vi "computeSetpoints.vi"(9 "Mdot":dbl, 10 "OffCentre":dbl, 11 "MFCsIn":T1[](array[typedef])) -> (1 "InactiveMFCs 2":T1[](array[typedef]), 3 "ActiveMFCs":T1[](array[typedef]))   [LabVIEW 2016]
uses:
  MFCdescription.ctl
  MFCcapability.ctl
panel:
  out "mDotTotal":dbl
  out "mDots":dbl[](array[numeric])
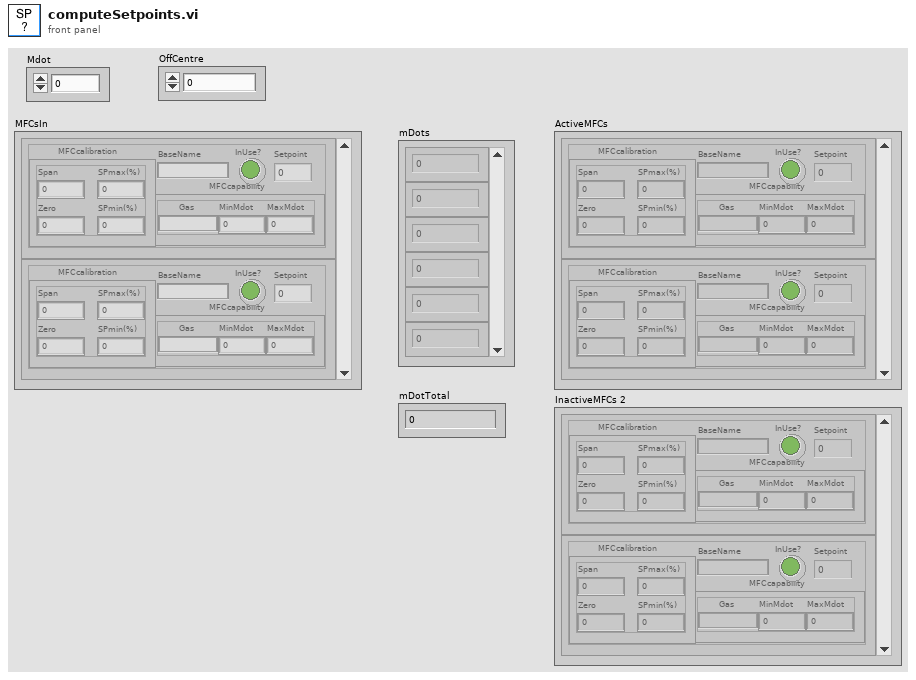
[diagram p1: front panel]
types:
  T1 = typedef "MFCdescription.ctl" = cluster{"BaseName":string, "MFCcalibration":cluster{"Span":dbl, "Zero":dbl, "SPmin(%)":dbl, "SPmax(%)":dbl}, "MFCcapability":T2, "InUse?":bool, "Setpoint":dbl}
  T2 = typedef "MFCcapability.ctl" = cluster{"Gas":string, "MinMdot":dbl, "MaxMdot":dbl}
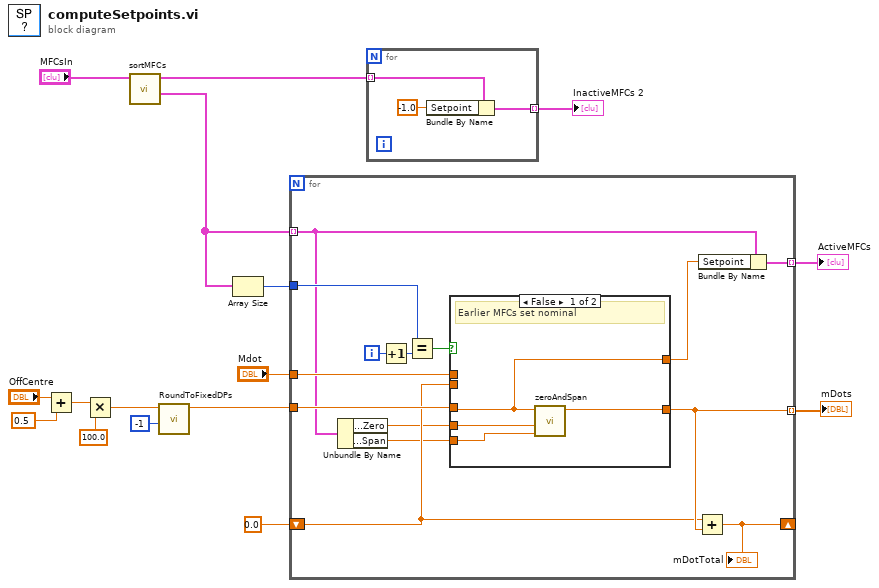
[diagram p0: block diagram]
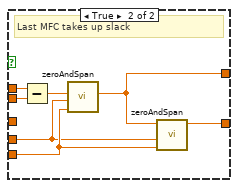
[diagram p2: hidden frame]
diagram:
  n1 = Add(x="OffCentre", y=0.5) -> (x+y=w5:dbl)
  n2 = Multiply(x=w5, y=100.0) -> (x*y=w2:dbl)
  n3 = call "sortMFCs.vi"("MFCs"="MFCsIn") -> ("InUseMFCsascending"=w10:T1[], "notInUseMFCsascending"=w7:T1[])  [unwired: 7 in, 2 out]
  n4 = call "RoundToFixedDPs.vi"("Power of ten"=-1, "Number to round"=w2) -> ("Rounded number"=w4:dbl)  [unwired: 8 in, 1 out]
  n5 = Array Size(array=w10) -> (size(s)=w9:i32)
  n6 = for {
    tunnel: w4 -> [w29]
    tunnel: "Mdot" -> [w28]
    tunnel: [w30] -> w13 mode=indexing
    shift-right: [w24] -> _
    shift-left: 0.0 -> [w27]
    tunnel: w10 -> [w19] mode=indexing
    tunnel: w9 -> [w22]
    tunnel: [w17] -> w8 mode=indexing
    i -> [w23]
    n7 = Unbundle By Name(w19) -> ("MFCcalibration.Zero"=w26:dbl, "MFCcalibration.Span"=w25:dbl)
    n8 = Increment(x=w23) -> (x+1=w21:i32)
    n9 = Equal?(x=w22, y=w21) -> (x = y?=w20:bool)
    n10 = case shown="False" w20 {
      tunnel: w29 -> [w31 _]
      tunnel: [w34 w36] -> w30
      tunnel: w28 -> [_ w41]
      tunnel: w27 -> [_ w40]
      tunnel: w26 -> [w33 w37]
      tunnel: w25 -> [w32 w38]
      tunnel: [w31 w35] -> w18
      frame False {
        # "Earlier MFCs set nominal"
        n11 = call "zeroAndSpan.vi"("spanValue"=w32, "zeroValue"=w33, "MeasuredPercent"=w31) -> ("calibratedOutput"=w34:dbl)  [unwired: 6 in, 2 out]
      }
      frame True {
        # "Last MFC takes up slack"
        n12 = Subtract(x=w41, y=w40) -> (x-y=w39:dbl)
        n13 = call "zeroAndSpan.vi"("spanValue"=w38, "zeroValue"=w37, "DesiredValue"=w39) -> ("PercentToSet"=w35:dbl)  [unwired: 6 in, 2 out]
        n14 = call "zeroAndSpan.vi"("spanValue"=w38, "zeroValue"=w37, "MeasuredPercent"=w35) -> ("calibratedOutput"=w36:dbl)  [unwired: 6 in, 2 out]
      }
    }
    n15 = Add(x=w27, y=w30) -> (x+y=w24:dbl)
    "mDotTotal" <- w24
    n16 = Bundle By Name(cluster=w19, "Setpoint"=w18) -> (w17:T1)
  }
  "mDots" <- w13
  "ActiveMFCs" <- w8
  n17 = for {
    tunnel: w7 -> [w44] mode=indexing
    tunnel: [w42] -> w6 mode=indexing
    n18 = Bundle By Name(cluster=w44, "Setpoint"=-1.0) -> (w42:T1)
  }
  "InactiveMFCs 2" <- w6
